vi "Handle Failure Action.vi"(7 "UDP Port":refnum<k16>, 8 "error in (no error)":errorcluster, 9 "Created New":bool, 10 "Assert FA SEQ":refnum<queue>, 11 "Assert Message in":T1) -> (0 "error out":errorcluster, 3 "Assert Message out":T1)   [LabVIEW 2016, in "Assert API Components.lvlib" / "Log Assert Core.lvlib"]
doc: "If an assert fails then get the current information from the single element queue for the assert failure action, and then calls the appropriate class for the failure action."
uses:
  Log Assert Core.lvlib
  Message Data.ctl
  VI References.ctl
  Failure Actions/Abort Application/Abort Application.lvclass
  D:/Work/Projects/Actor_Assert_API/Assert API Components/Log Assert Core Components/Failure Actions/Fail Action Base.lvclass
  Failure Actions/Log To File/Log To File.lvclass
  Failure Actions/Fail Action Base.lvclass
  Failure Actions/Pause Application/Pause Application.lvclass
  Assert API Components.lvlib
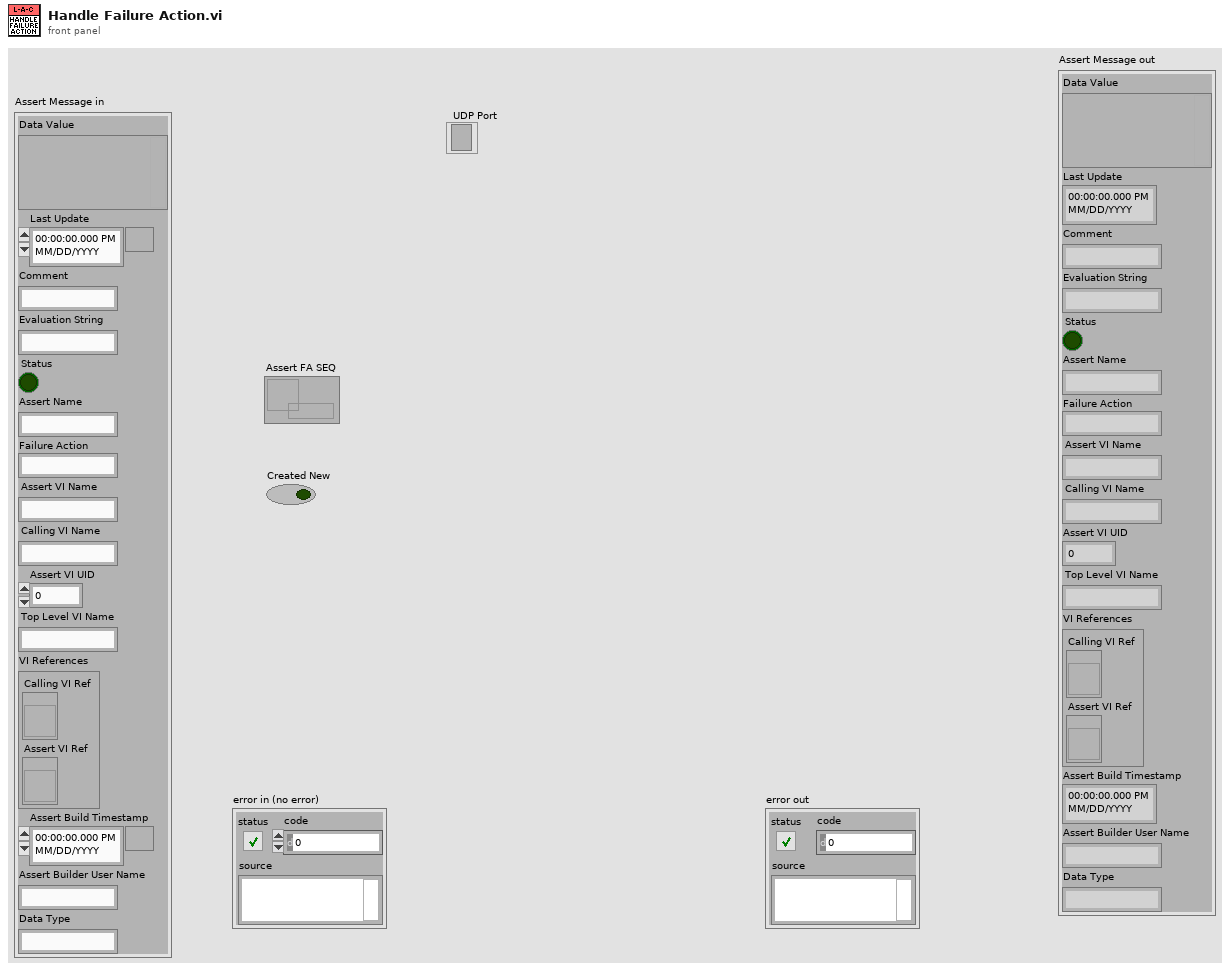
[diagram p1: front panel]
types:
  T1 = typedef "Assert API Components.lvlib/Message Data.ctl" = cluster{"Data Value":variant, "Last Update":timestamp, "Comment":string, "Evaluation String":string, "Status":bool, "Assert Name":string, "Failure Action":string, "Assert VI Name":string, "Calling VI Name":string, "Assert VI UID":i32, "Top Level VI Name":string, "VI References":T2, "Assert Build Timestamp":timestamp, "Assert Builder User Name":string, "Data Type":string}
  T2 = typedef "Assert API Components.lvlib/VI References.ctl" = cluster{"Calling VI Ref":refnum<vi>, "Assert VI Ref":refnum<vi>}
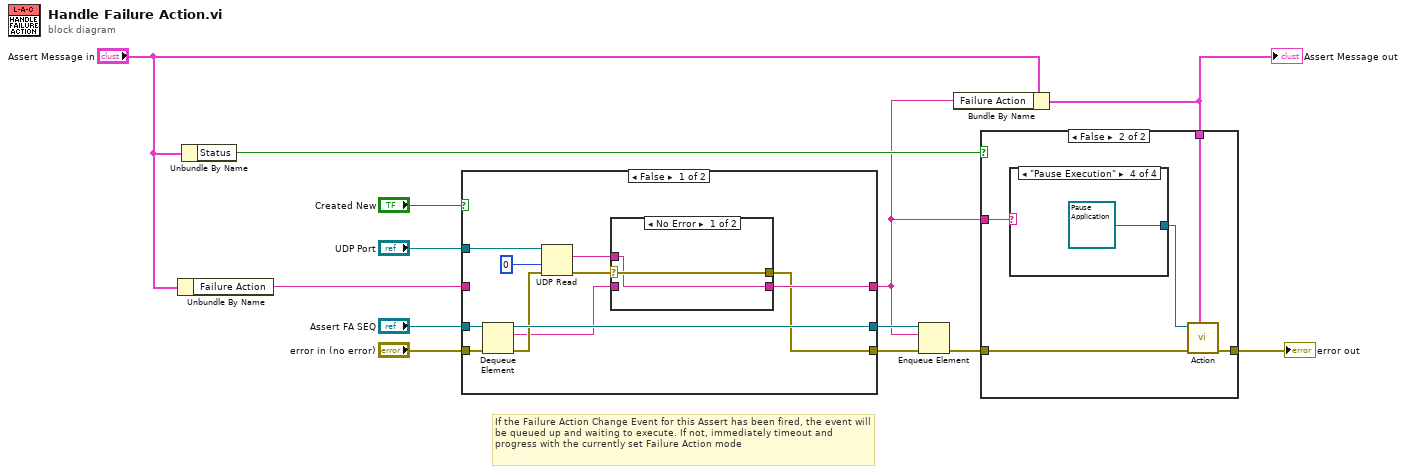
[diagram p0: block diagram]
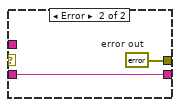
[diagram p2: hidden frame]
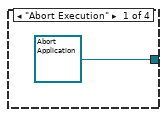
[diagram p5: hidden frame]
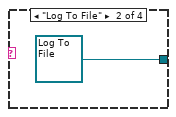
[diagram p6: hidden frame]
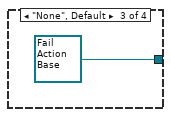
[diagram p7: hidden frame]
diagram:
  # "If the Failure Action Change Event for this Assert has been fired, the event will be queued up and waiting to execute. If not, immediately timeout and progress with the currently set Failure Action mode"
  n1 = Unbundle By Name("Assert Message in") -> ("Failure Action"=w10:string)
  n2 = Unbundle By Name("Assert Message in") -> ("Status"=w9:bool)
  n3 = case shown="False" "Created New" {
    tunnel: [w20 w29] -> w6
    tunnel: "UDP Port" -> [w18 _]
    tunnel: "Assert FA SEQ" -> [w24 w30]
    tunnel: "error in (no error)" -> [w23 w31]
    tunnel: [w16 w31] -> w12
    tunnel: [w22 w30] -> w11
    tunnel: w10 -> [_ w29]
    frame False {
      n4 = Dequeue Element(queue=w24, error in (no error)=w23) -> (queue out=w22:refnum<queue>, element=w15:string, error out=w21:errorcluster)  [unwired: 1 in, 1 out]
      n5 = UDP Read(connection ID=w18, timeout ms (25000)=0, 8:w21) -> (data out=w14:string, error out=w19:errorcluster)  [unwired: 1 in, 3 out]
      n6 = case shown="No Error" w19 {
        selector: w19 -> [w26 _]
        tunnel: [w25 w28] -> w20
        tunnel: [w26 w27] -> w16
        tunnel: w15 -> [_ w28]
        tunnel: w14 -> [w25 _]
        frame No Error {
        }
        frame Error {
          w27 = errorcluster {"status"=FALSE, "code"=0, "source"=""}  # error out
        }
      }
    }
    frame True {
      # "Takes the default failure action on the first call but thereafter looks in the SEQ"
    }
  }
  n7 = Enqueue Element(queue=w11, element=w6, error in (no error)=w12) -> (error out=w5:errorcluster)  [unwired: 1 in, 2 out]
  n8 = Bundle By Name(cluster="Assert Message in", "Failure Action"=w6) -> (w4:T1)
  "Assert Message out" <- w4
  n9 = case shown="False" w9 {
    tunnel: w6 -> [_ w37]
    tunnel: w5 -> [w32 w36]
    tunnel: w4 -> [_ w34]
    tunnel: [w32 w33] -> w3
    frame True {
      # "Assert passed - no action"
    }
    frame False {
      n10 = case shown="\"Pause Execution\"" w37 {
        tunnel: [refnum<class "Abort Application.lvclass"> refnum ("Assert API Components.lvlib:Log Assert Core.lvlib:Abort Application.lvclass") refnum<class "Log To File.lvclass"> refnum ("Assert API Components.lvlib:Log Assert Core.lvlib:Log To File.lvclass") refnum<class "Fail Action Base.lvclass"> refnum ("Assert API Components.lvlib:Log Assert Core.lvlib:Fail Action Base.lvclass") refnum<class "Pause Application.lvclass"> refnum ("Assert API Components.lvlib:Log Assert Core.lvlib:Pause Application.lvclass")] -> w35
        frame "Abort Execution" {
        }
        frame "Log To File" {
        }
        frame "None", Default {
        }
        frame "Pause Execution" {
        }
      }
      n11 = call-dynamic "Action.vi"("Assert Message"=w34, "error in (no error)"=w36, "Fail Action Base in"=w35) -> ("error out"=w33:errorcluster)  [unwired: 8 in]
    }
  }
  "error out" <- w3
